vi "LearnVI.vi"() -> ()   [LabVIEW 2015]
uses:
  StateType.ctl
  <vilib>/FPGAPlugInAG/PXI-7841R/niLvFpga_Open_PXI-7841R.vi
  <vilib>/rvi/interface/common/dynamic/niFpgaDynamicAddResources.vi
  <vilib>/FPGAPlugInAG/Dynamic/niLvFpga_Run_Dynamic.vi
  <vilib>/Utility/error.llb/Error Cluster From Error Code.vi
  <vilib>/rvi/errors/niLvFpgaAdjustHostInterfaceError.vi
  <vilib>/FPGAPlugInAG/Dynamic/niLvFpga_Close_Dynamic.vi
  <vilib>/rvi/interface/nirviOpenFPGA/nirviOpenFPGA.xnode
  FPGA Bitfiles/PerceptronLearni_FPGATarget_Main_ZilKqRoJ7Xc.lvbitx
  Main.vi
  <vilib>/rvi/interface/nirviMethod/nirviMethod.xnode
  <vilib>/rvi/interface/nirviReadWriteControl/nirviReadWriteControl.xnode
  <vilib>/rvi/interface/nirviCloseFPGA/nirviCloseFPGA.xnode
  <vilib>/rvi/interface/Simulation/niFpgaSimulationCallBeginRW.vi
  NiFpgaLv.dll
panel:
  out "Coefficients":u16[](array[numeric])
  in  "Current Number":i8
  in  "STOP":bool
  in  "Iteration Number":u32
  in  "State":T1
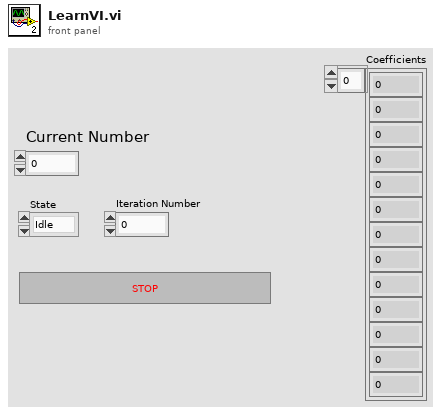
[diagram p1: front panel]
types:
  T1 = typedef "StateType.ctl" = enum16{"Idle", "Learning", "Read"}
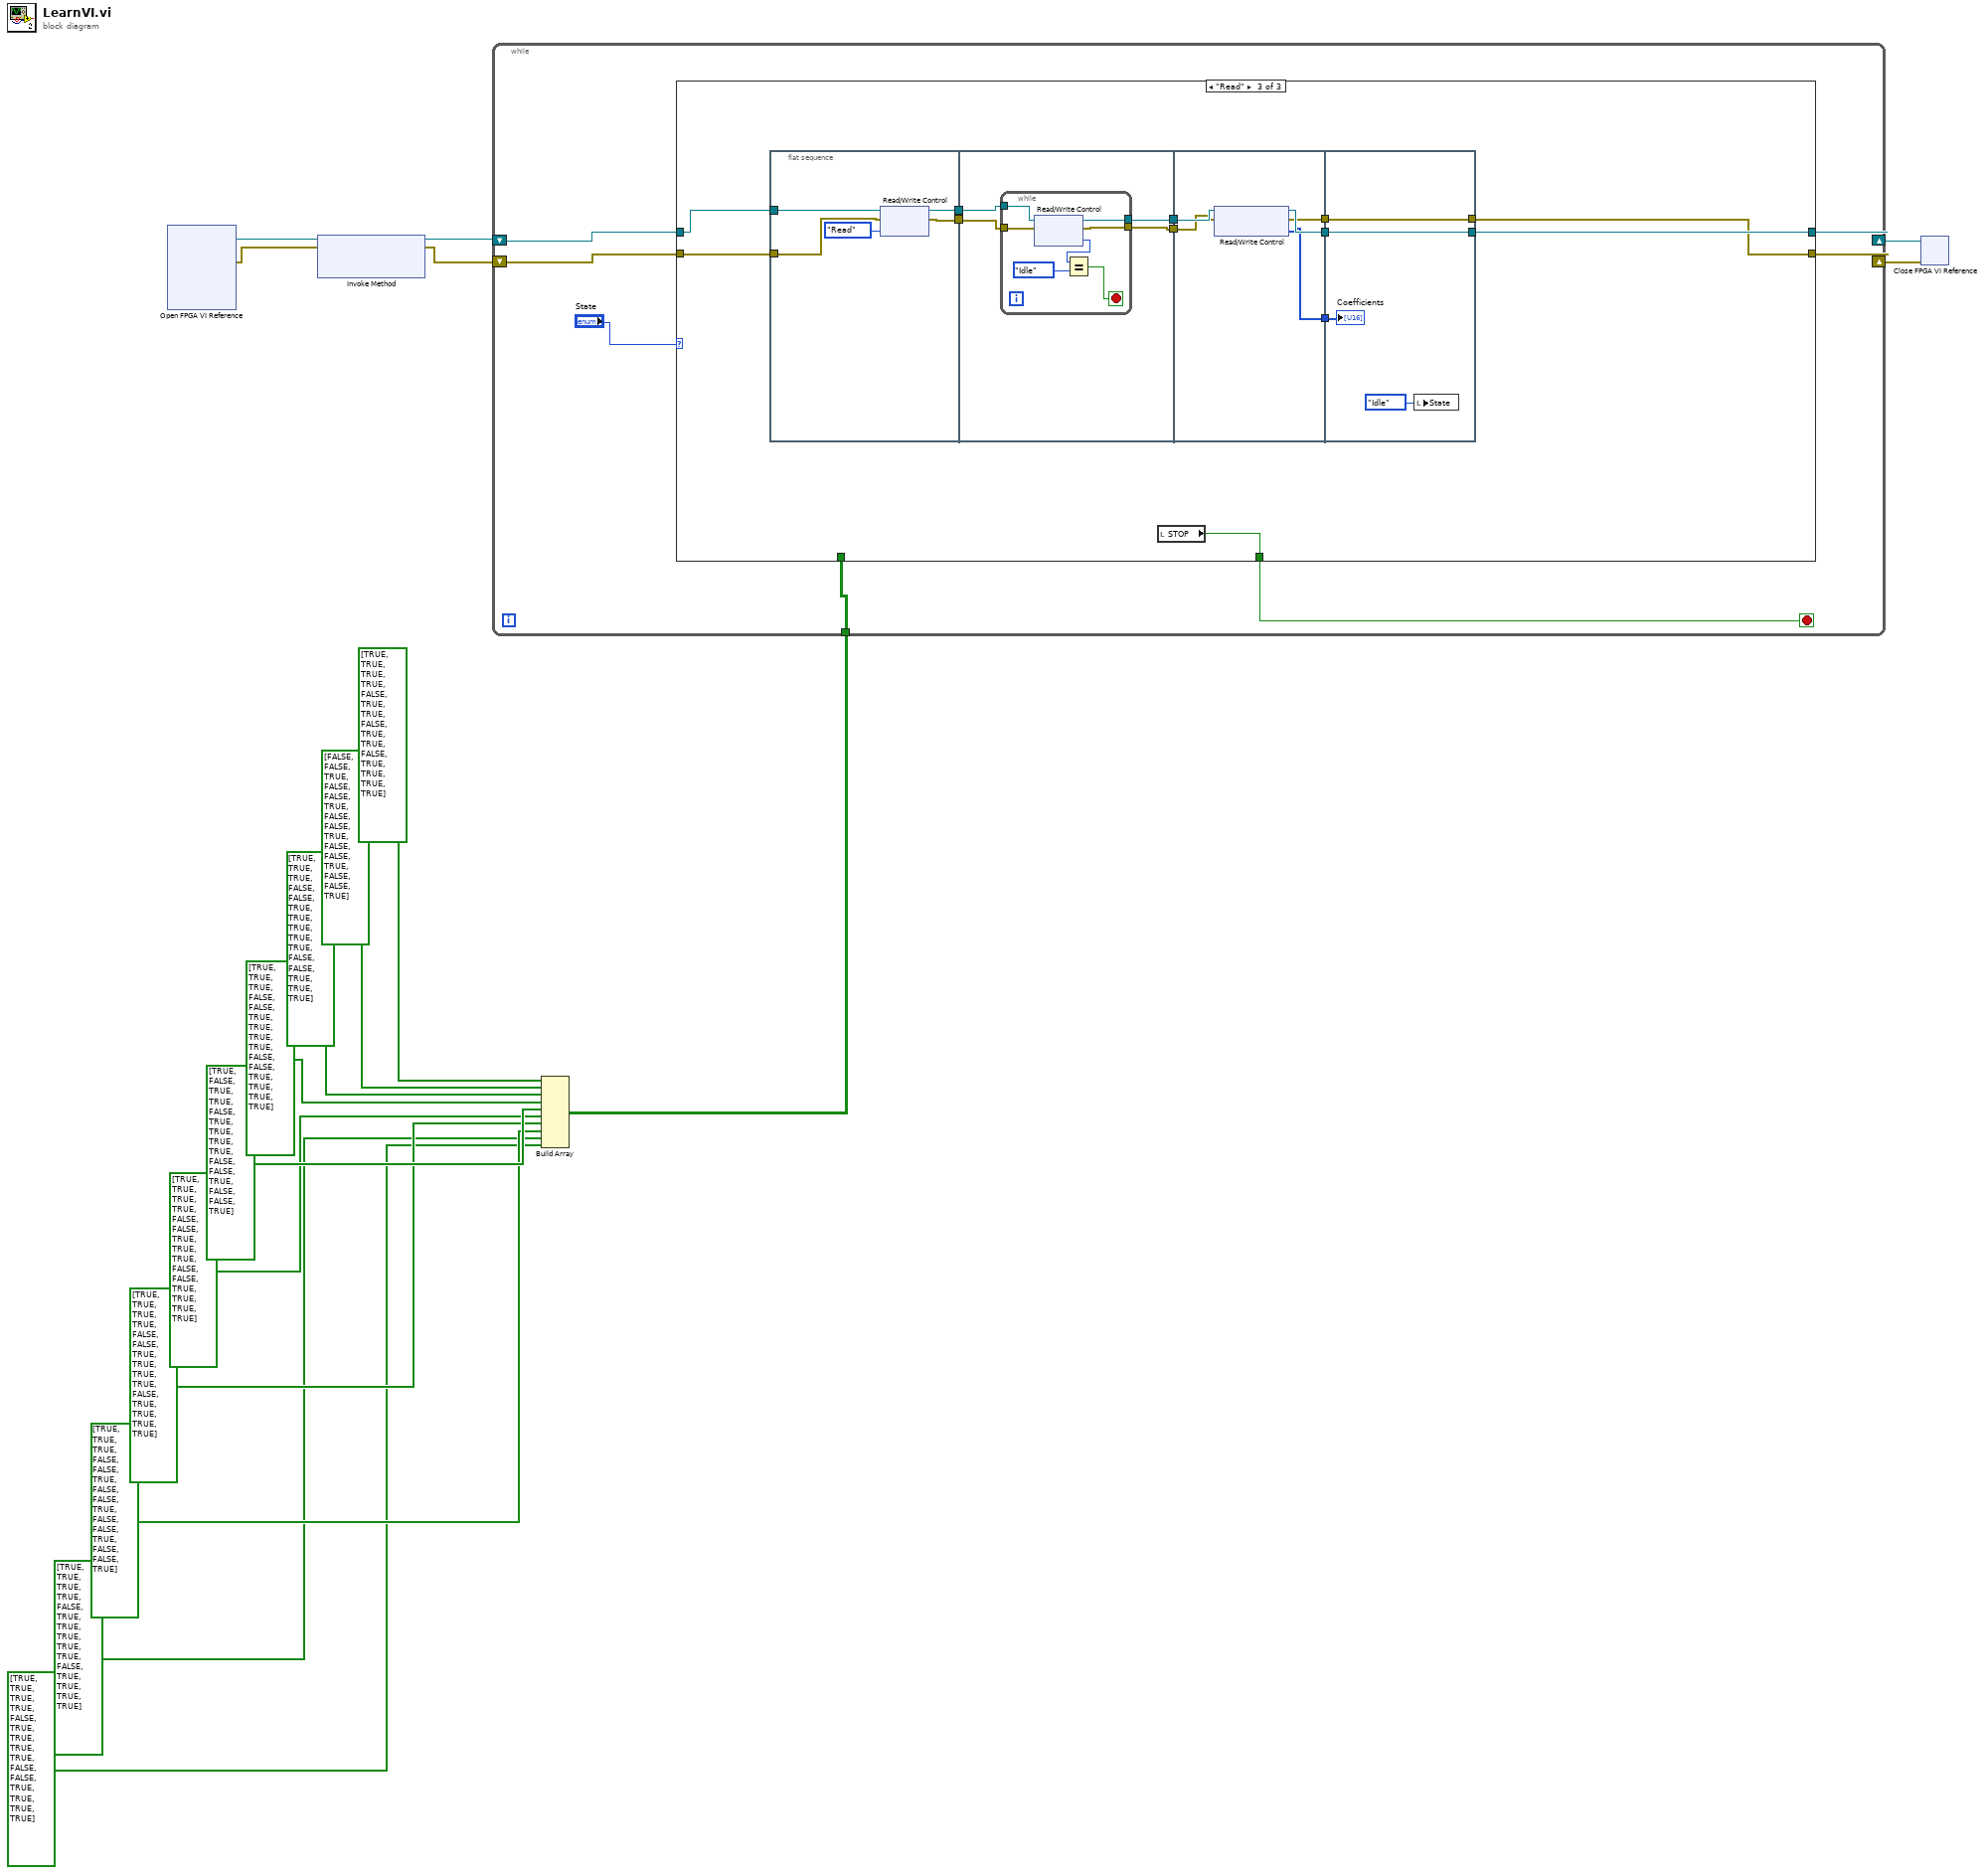
[diagram p0: block diagram]
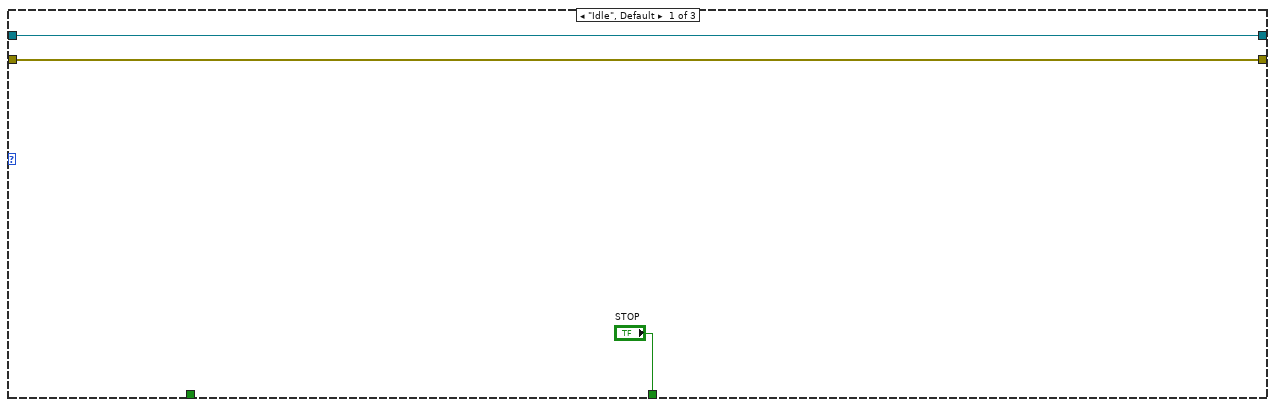
[diagram p2: hidden frame]
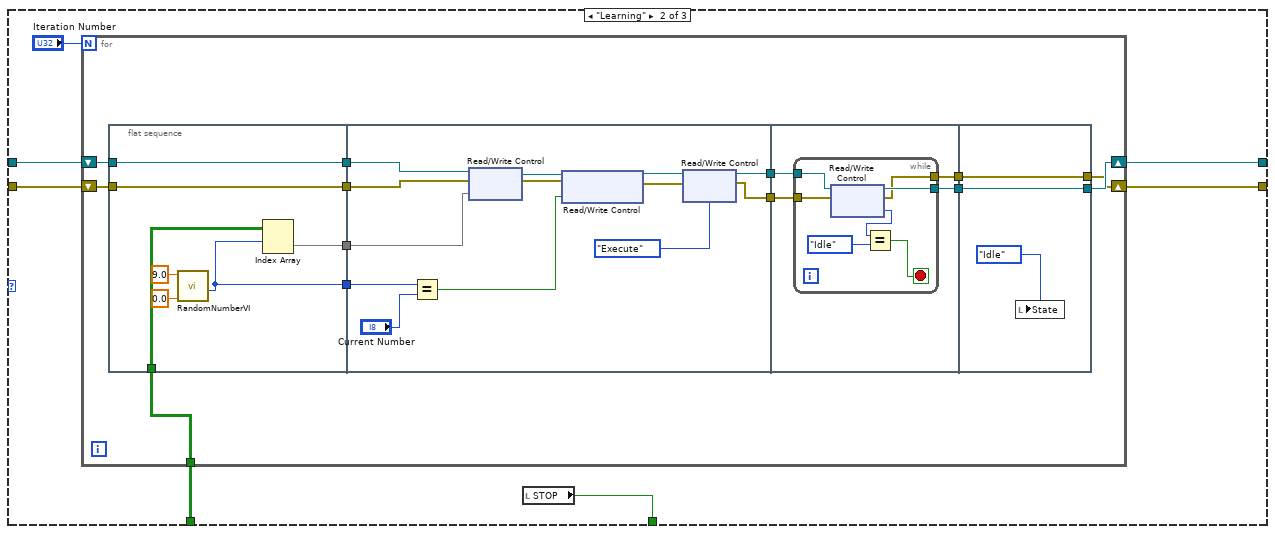
[diagram p3: hidden frame]
diagram:
  n1 = xnode "Open FPGA VI Reference"() -> ("FPGA VI Reference Out"=w4:refnum<k20>, "error out"=w3:errorcluster)  [unwired: 2 in]
  n2 = xnode "Invoke Method"("FPGA VI Reference In"=w4, "error in"=w3) -> ("FPGA VI Reference Out"=w2:refnum<k20>, "error out"=w1:errorcluster)  [unwired: 1 in]
  n3 = Build Array(bool[] [TRUE, TRUE, TRUE, TRUE, FALSE, TRUE, TRUE, FALSE, TRUE, TRUE, FALSE, TRUE, TRUE, TRUE, TRUE], bool[] [FALSE, FALSE, TRUE, FALSE, FALSE, TRUE, FALSE, FALSE, TRUE, FALSE, FALSE, TRUE, FALSE, FALSE, TRUE], bool[] [TRUE, TRUE, TRUE, FALSE, FALSE, TRUE, TRUE, TRUE, TRUE, TRUE, FALSE, FALSE, TRUE, TRUE, TRUE], bool[] [TRUE, TRUE, TRUE, FALSE, FALSE, TRUE, TRUE, TRUE, TRUE, FALSE, FALSE, TRUE, TRUE, TRUE, TRUE], bool[] [TRUE, FALSE, TRUE, TRUE, FALSE, TRUE, TRUE, TRUE, TRUE, FALSE, FALSE, TRUE, FALSE, FALSE, TRUE], bool[] [TRUE, TRUE, TRUE, TRUE, FALSE, FALSE, TRUE, TRUE, TRUE, FALSE, FALSE, TRUE, TRUE, TRUE, TRUE], bool[] [TRUE, TRUE, TRUE, TRUE, FALSE, FALSE, TRUE, TRUE, TRUE, TRUE, FALSE, TRUE, TRUE, TRUE, TRUE], bool[] [TRUE, TRUE, TRUE, FALSE, FALSE, TRUE, FALSE, FALSE, TRUE, FALSE, FALSE, TRUE, FALSE, FALSE, TRUE], bool[] [TRUE, TRUE, TRUE, TRUE, FALSE, TRUE, TRUE, TRUE, TRUE, TRUE, FALSE, TRUE, TRUE, TRUE, TRUE], bool[] [TRUE, TRUE, TRUE, TRUE, FALSE, TRUE, TRUE, TRUE, TRUE, FALSE, FALSE, TRUE, TRUE, TRUE, TRUE]) -> (w7:bool[][])
  n4 = while {
    tunnel: w7 -> [w23]
    shift-right: [w19] -> w6
    shift-left: w2 -> [w21]
    shift-right: [w18] -> w5
    shift-left: w1 -> [w20]
    stop <- w24 stop-if-true
    n5 = case shown="\"Read\"" "State" {
      tunnel: ["STOP" w28 w82] -> w24
      tunnel: w23 -> [_ w33 _]
      tunnel: w21 -> [w26 w32 w93]
      tunnel: w20 -> [w25 w31 w92]
      tunnel: [w26 w30 w87] -> w19
      tunnel: [w25 w29 w86] -> w18
      frame "Idle", Default {
      }
      frame "Learning" {
        n6 = for {
          N: "Iteration Number" -> [_]
          tunnel: w33 -> [w47]
          shift-right: [w38] -> w30
          shift-left: w32 -> [w45]
          shift-right: [w37] -> w29
          shift-left: w31 -> [w43]
          n7 = flat-sequence {
            tunnel: w47 -> [w52]
            tunnel: [w51] -> w46
            tunnel: w45 -> [w51]
            tunnel: [w50] -> w44
            tunnel: w43 -> [w50]
            tunnel: [w49] -> w42
            tunnel: [w48] -> w41
            tunnel: w46 -> [w67]
            tunnel: w44 -> [w66]
            tunnel: w42 -> [w65]
            tunnel: w41 -> [w62]
            tunnel: [w57] -> w40
            tunnel: [w56] -> w39
            tunnel: w40 -> [w71]
            tunnel: w39 -> [w70]
            tunnel: [w69] -> w36
            tunnel: [w68] -> w35
            tunnel: [w80] -> w37
            tunnel: [w81] -> w38
            tunnel: w36 -> [w81]
            tunnel: w35 -> [w80]
            frame #0 {
              n8 = call "RandomNumberVI.vi"("Lower Limit"=0.0, "Upper Limit"=9.0) -> ("Random Number I8"=w48:i8)  [unwired: 6 in, 3 out]
              n9 = Index Array(array=w52, index (row)=w48) -> (element=w49:bool[])  [unwired: 1 in]
            }
            frame #1 {
              n10 = Equal?(x=w62, y="Current Number") -> (x = y?=w60:bool)
              n11 = xnode "Read/Write Control"("FPGA VI Reference In"=w67, "error in"=w66, "Data"=w65) -> ("FPGA VI Reference Out"=w64:refnum<k20>, "error out"=w63:errorcluster)
              n12 = xnode "Read/Write Control"("FPGA VI Reference In"=w64, "error in"=w63, "Right Result"=w60) -> ("FPGA VI Reference Out"=w59:refnum<k20>, "error out"=w58:errorcluster)
              n13 = xnode "Read/Write Control"("FPGA VI Reference In"=w59, "error in"=w58, "State"=enum16{"Read", "Idle", "Execute", "End"}."Execute") -> ("FPGA VI Reference Out"=w57:refnum<k20>, "error out"=w56:errorcluster)
            }
            frame #2 {
              n14 = while {
                tunnel: w71 -> [w78]
                tunnel: w70 -> [w77]
                tunnel: [w74] -> w69
                tunnel: [w73] -> w68
                stop <- w75 stop-if-true
                n15 = xnode "Read/Write Control"("FPGA VI Reference In"=w78, "error in"=w77) -> ("FPGA VI Reference Out"=w74:refnum<k20>, "error out"=w73:errorcluster, "State"=w76:enum16{"Read", "Idle", "Execute", "End"})
                n16 = Equal?(x=w76, y=enum16{"Read", "Idle", "Execute", "End"}."Idle" ("State")) -> (x = y?=w75:bool)
              }
            }
            frame #3 {
              n17 = local write "State"(StateType."Idle" ("State")) -> ()
            }
          }
        }
        n18 = local read "STOP"() -> (w28:bool)
      }
      frame "Read" {
        n19 = flat-sequence {
          tunnel: w93 -> [w97]
          tunnel: w92 -> [w96]
          tunnel: [w95] -> w91
          tunnel: [w94] -> w90
          tunnel: w91 -> [w102]
          tunnel: w90 -> [w101]
          tunnel: [w100] -> w89
          tunnel: [w99] -> w88
          tunnel: w89 -> [w114]
          tunnel: w88 -> [w113]
          tunnel: [w112] -> w85
          tunnel: [w111] -> w84
          tunnel: [w110] -> w83
          tunnel: w85 -> [w118]
          tunnel: w84 -> [w117]
          tunnel: w83 -> [w115]
          tunnel: [w118] -> w87
          tunnel: [w117] -> w86
          frame #0 {
            n20 = xnode "Read/Write Control"("FPGA VI Reference In"=w97, "error in"=w96, "State"=enum16{"Read", "Idle", "Execute", "End"}."Read") -> ("FPGA VI Reference Out"=w95:refnum<k20>, "error out"=w94:errorcluster)
          }
          frame #1 {
            n21 = while {
              tunnel: w102 -> [w109]
              tunnel: w101 -> [w103]
              tunnel: [w106] -> w100
              tunnel: [w105] -> w99
              stop <- w107 stop-if-true
              n22 = xnode "Read/Write Control"("FPGA VI Reference In"=w109, "error in"=w103) -> ("FPGA VI Reference Out"=w106:refnum<k20>, "error out"=w105:errorcluster, "State"=w108:enum16{"Read", "Idle", "Execute", "End"})
              n23 = Equal?(x=w108, y=enum16{"Read", "Idle", "Execute", "End"}."Idle" ("State")) -> (x = y?=w107:bool)
            }
          }
          frame #2 {
            n24 = xnode "Read/Write Control"("FPGA VI Reference In"=w114, "error in"=w113) -> ("FPGA VI Reference Out"=w112:refnum<k20>, "error out"=w111:errorcluster, "Coefficients"=w110:u16[])
          }
          frame #3 {
            n25 = local write "State"(StateType."Idle" ("State")) -> ()
            "Coefficients" <- w115
          }
        }
        n26 = local read "STOP"() -> (w82:bool)
      }
    }
  }
  n27 = xnode "Close FPGA VI Reference"("FPGA VI Reference In"=w6, "error in"=w5) -> ()  [unwired: 1 out]
